vi "validDataString.vi"(8 "error in (no error)":errorcluster, 10 "value in":string, 11 "data type":T1) -> (0 "error out":errorcluster, 2 "value out":string, 3 "Valid":bool)   [LabVIEW 2013]
uses:
  <vilib>/NI/Tag Bus/tag/Data Type.ctl
  <vilib>/regexp/Match Regular Expression.xnode
  <vilib>/NI/Tag Bus/tag/tag descriptor.lvclass
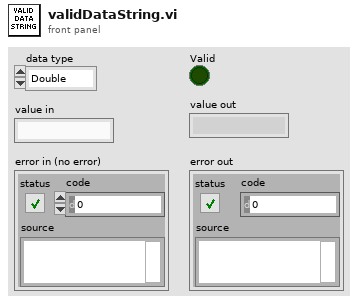
[diagram p1: front panel]
types:
  T1 = typedef "tag bus.lvlib/tag descriptor.lvclass/Data Type.ctl" = enum16{"Double", "Single", "I64", "I32", "I16", "I8", "U64", "U32", "U16", "U8", "Boolean", "String", "Array of Double", "Array of Single", "Array of I64", "Array of I32", "Array of I16", "Array of I8", "Array of U64", "Array of U32", "Array of U16", "Array of U8", "Array of Boolean", "Array of String"}
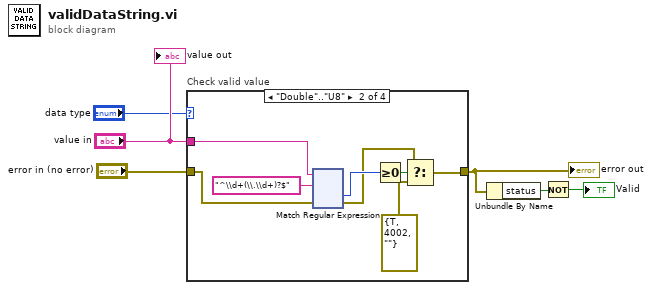
[diagram p0: block diagram]
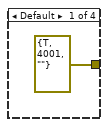
[diagram p2: hidden frame]
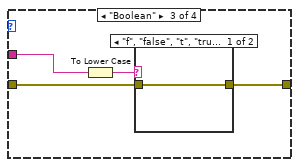
[diagram p3: hidden frame]
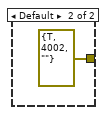
[diagram p4: hidden frame]
diagram:
  n1 = case "Check valid value" shown="\"Double\"..\"U8\"" "data type" {
    tunnel: "value in" -> [_ w13 w132 _]
    tunnel: "error in (no error)" -> [_ w10 w130 w136]
    tunnel: [errorcluster {"status"=TRUE, "code"=4001, "source"=""} ("error out") w11 w131 w136] -> w4
    frame Default {
    }
    frame "Double".."U8" {
      n2 = xnode "Match Regular Expression"("input string"=w13, "regular expression"="^\\d+(\\.\\d+)?$", "error in"=w10) -> ("offset past match"=w14:i32, "error out"=w9:errorcluster)  [unwired: 3 in, 3 out]
      n3 = Greater Or Equal To 0?(x=w14) -> (x >= 0?=w8:bool)
      n4 = Select(t=w9, s=w8, f=errorcluster {"status"=TRUE, "code"=4002, "source"=""} ("error out")) -> (s? t:f=w11:errorcluster)
    }
    frame "Boolean" {
      n5 = To Lower Case(string=w132) -> (all lower case string=w133:string)
      n6 = case shown="\"f\", \"false\", \"t\", \"true\"" w133 {
        tunnel: [w134 errorcluster {"status"=TRUE, "code"=4002, "source"=""} ("error out")] -> w131
        tunnel: w130 -> [w134 _]
        frame "f", "false", "t", "true" {
        }
        frame Default {
        }
      }
    }
    frame "String" {
    }
  }
  "error out" <- w4
  n7 = Unbundle By Name(w4) -> ("status"=w3:bool)
  n8 = Not(x=w3) -> (.not. x?=→"Valid":bool)
  "value out" <- "value in"
